vi "Append Tabs To String Front.vi"(4 "TabCount(4)":i32=4, 5 "Str in":string="NEVSTOP-MemBuffer.lvlib:memBuffer.lvclass:replace memory subs") -> (2 "Str out":string="replace memory subs")   [LabVIEW 2017]
doc: "Inserts TabCount tabs at the start of every line of Str in, so a block of text can be indented."
uses:
  Configuration/Ini/ini_configuration.lvlib
  _openG/_reuse_openG.lvlib
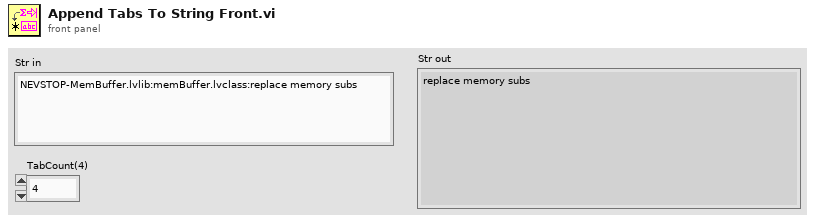
[diagram p1: front panel]
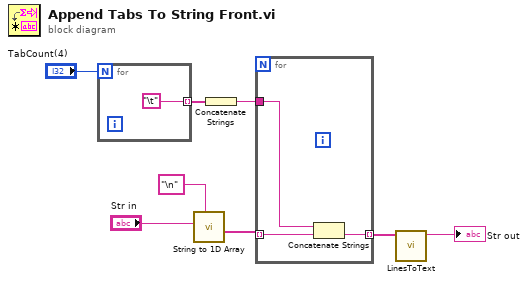
[diagram p0: block diagram]
diagram:
  n1 = for {
    N: "TabCount(4)" -> [_]
    tunnel: ["\t"] -> w4 mode=indexing
  }
  n2 = call "String to 1D Array.vi"("delimiter (Tab)"="\n", "string"="Str in") -> ("Array of Strings"=w2:string[])  [unwired: 9 in]
  n3 = Concatenate Strings(w4) -> (w3:string)
  n4 = for {
    tunnel: [w11] -> w8 mode=indexing
    tunnel: w2 -> [w12] mode=indexing
    tunnel: w3 -> [w10]
    n5 = Concatenate Strings(w10, w12) -> (w11:string)
  }
  n6 = call "LinesToText.vi"("Lines"=w8) -> ("string"=→"Str out":string)  [unwired: 9 in, 1 out]
